vi "Actor Core.vi"(8 "error in":errorcluster, 11 "Simulated Evaporative Cooler":refnum<class "Simulated Evaporative Cooler.lvclass">) -> (0 "error out":errorcluster, 3 "Actor out":refnum<class "Actor.lvclass">)   [LabVIEW 2025, in "Simulated Evaporative Cooler.lvclass"]
doc: "This is Actor Core.vi, the main message handling loop for Actors. An actor usually just sits in this loop and processes messages as they arrive. Any error returned by the message Do.vi call will stop the loop, with error code 43 as the canonical signal to stop with no error sent to caller. Descendants may override that in Handle Error.vi."
uses:
  Simulated Evaporative Cooler.lvclass
  <vilib>/ActorFramework/Actor/Actor.lvclass
  Simulation Data_Global.vi
  Evaporative Cooler/Evaporative Cooler/Evaporative Cooler.lvclass
panel:
  out "stop signal":bool
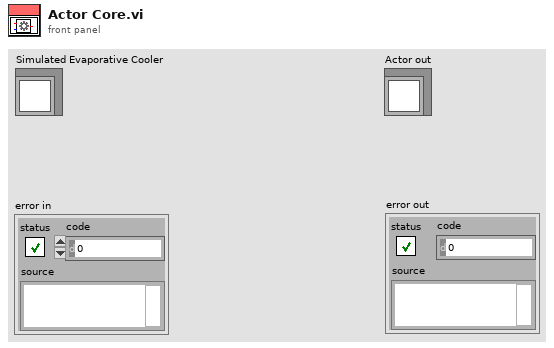
[diagram p1: front panel]
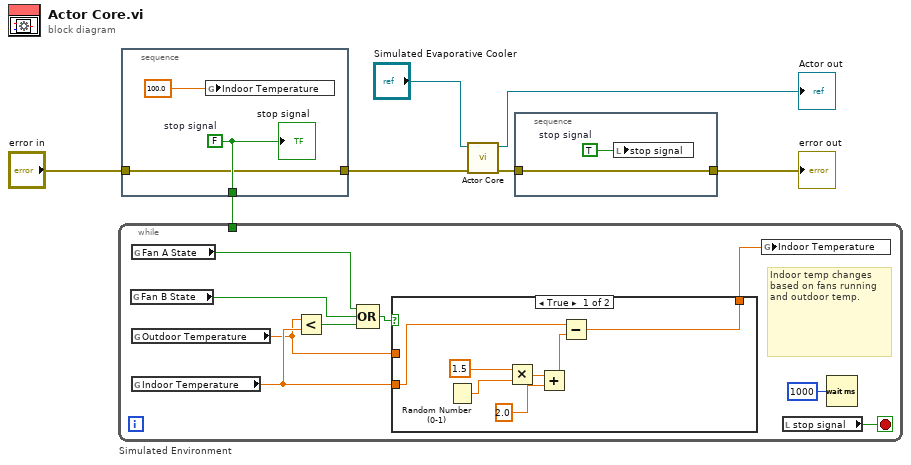
[diagram p0: block diagram]
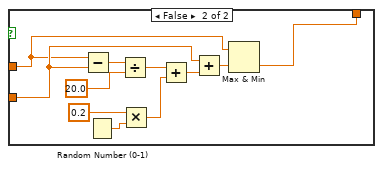
[diagram p2: hidden frame]
diagram:
  n1 = stacked-sequence {
    tunnel: [w10] -> w7
    tunnel: [w9] -> w4
    tunnel: "error in" -> [w9]
    frame #0 {
      w10 = FALSE  # stop signal
      n2 = global write "Simulation Data_Global.vi" "Indoor Temperature"(100.0 ("Temperature")) -> ()
      "stop signal" <- w10
    }
  }
  n3 = while "Simulated Environment" {
    tunnel: w7 -> [_]
    stop <- w18 stop-if-true
    # "Indoor temp changes based on fans running and outdoor temp."
    n4 = global read "Simulation Data_Global.vi" "Fan B State"() -> (w12:bool)
    n5 = global read "Simulation Data_Global.vi" "Fan A State"() -> (w13:bool)
    n6 = global read "Simulation Data_Global.vi" "Outdoor Temperature"() -> (w14:dbl)
    n7 = global read "Simulation Data_Global.vi" "Indoor Temperature"() -> (w15:dbl)
    n8 = Less?(x=w14, y=w15) -> (x < y?=w16:bool)
    n9 = Compound Arithmetic op=OR(w13, w12, w16) -> (w19:bool)
    n10 = case shown="True" w19 {
      tunnel: w15 -> [w21 w29]
      tunnel: w14 -> [_ w28]
      tunnel: [w20 w27] -> w11
      frame True {
        n11 = Random Number (0-1)() -> (number: 0 to 1=w25:dbl)
        n12 = Multiply(x=1.5 ("y"), y=w25) -> (x*y=w24:dbl)
        n13 = Add(x=w24, y=2.0) -> (x+y=w22:dbl)
        n14 = Subtract(x=w21, y=w22) -> (x-y=w20:dbl)
      }
      frame False {
        n15 = Subtract(x=w28, y=w29) -> (x-y=w37:dbl)
        n16 = Random Number (0-1)() -> (number: 0 to 1=w33:dbl)
        n17 = Divide(x=w37, y=20.0) -> (x/y=w35:dbl)
        n18 = Multiply(x=0.2, y=w33) -> (x*y=w32:dbl)
        n19 = Add(x=w35, y=w32) -> (x+y=w31:dbl)
        n20 = Add(x=w29, y=w31) -> (x+y=w30:dbl)
        n21 = Max & Min(x=w28, y=w30) -> (min(x,y)=w27:dbl)  [unwired: 1 out]
      }
    }
    n22 = global write "Simulation Data_Global.vi" "Indoor Temperature"(w11) -> ()
    n23 = local read "stop signal"() -> (w18:bool)
    n24 = Wait (ms)(milliseconds to wait=u32 1000) -> ()  [unwired: 1 out]
  }
  n25 = call-parent "Actor Core.vi"("error in"=w4, "Evaporative Cooler"="Simulated Evaporative Cooler") -> ("error out"=w1:errorcluster, "Actor out"=→"Actor out":refnum<class "Actor.lvclass">)  [unwired: 8 in]
  n26 = stacked-sequence {
    tunnel: [w38] -> w2
    tunnel: w1 -> [w38]
    frame #0 {
      w39 = TRUE  # stop signal
      n27 = local write "stop signal"(w39) -> ()
    }
  }
  "error out" <- w2
